vi "PDFCreator Get Options.vi"(0 "PDFCreator._clsPDFCreator":refnum<k7>, 11 "error in (no error)":errorcluster) -> (4 "PDFCreator._clsPDFCreator 2":refnum<k7>, 8 "Options":T1, 15 "error out":errorcluster)   [LabVIEW 2010]
doc: "Jean-Marc Simard \nJanuary 6, 2010"
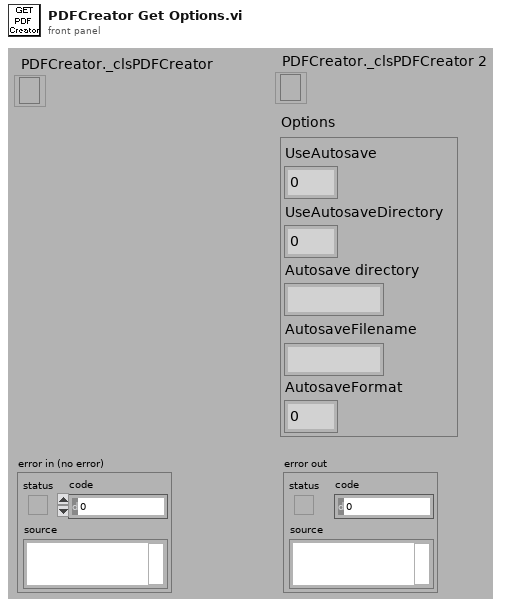
[diagram p1: front panel]
types:
  T1 = cluster{"UseAutosave":i32, "UseAutosaveDirectory":i32, "Autosave directory":string, "AutosaveFilename":string, "AutosaveFormat":i32}
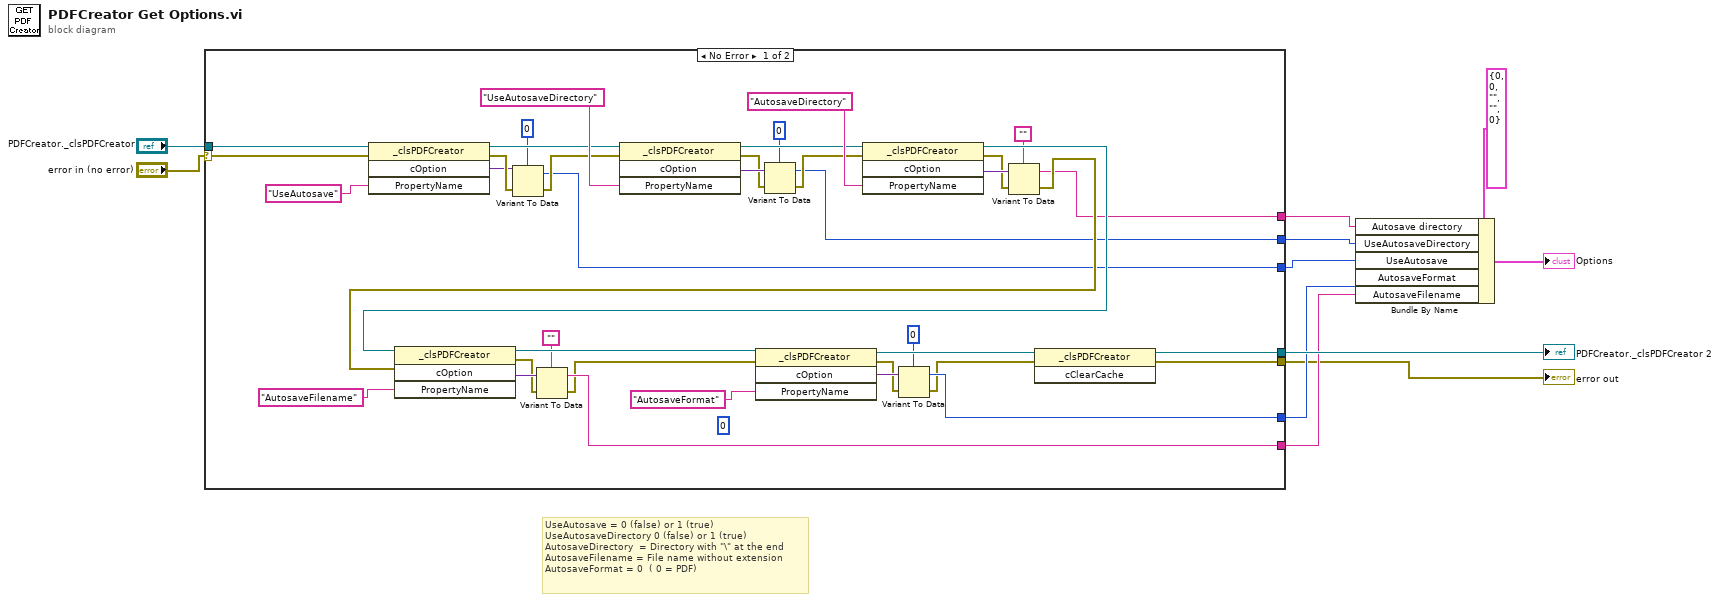
[diagram p0: block diagram]
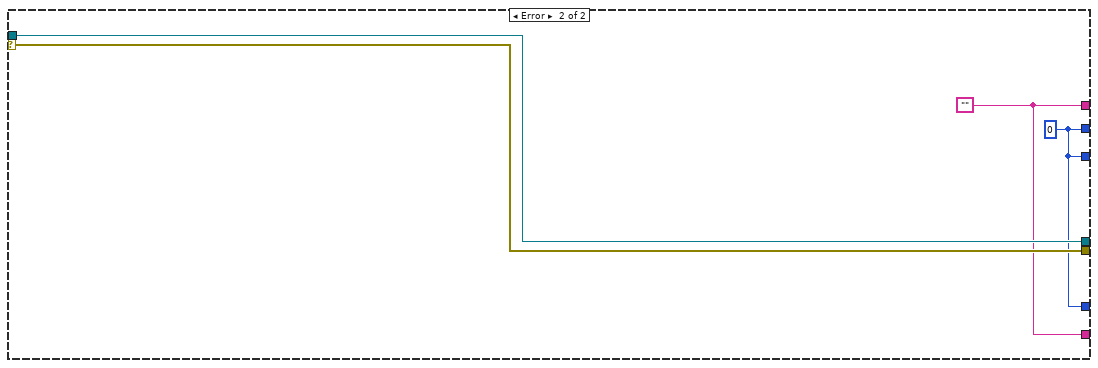
[diagram p2: hidden frame]
diagram:
  # "UseAutosave = 0 (false) or 1 (true)\nUseAutosaveDirectory 0 (false) or 1 (true)\nAutosaveDirectory  = Directory with \"\\\" at the end\nAutosaveFilename = File name without extension \nAutosaveFormat = 0  ( 0 = PDF)"
  n1 = case shown="No Error" "error in (no error)" {
    selector: "error in (no error)" -> [w39 w53]
    tunnel: [w22 w54] -> w11
    tunnel: [w21 w53] -> w1
    tunnel: "PDFCreator._clsPDFCreator" -> [w40 w54]
    tunnel: [w20 w52] -> w9
    tunnel: [w19 w51] -> w8
    tunnel: [w18 w51] -> w7
    tunnel: [w17 w51] -> w6
    tunnel: [w16 w52] -> w5
    frame No Error {
      (unwired) 0
      n2 = invoke class="_clsPDFCreator" method="cOption"(reference=w40, error in=w39, "PropertyName"="UseAutosave") -> (reference out=w48:refnum<k7>, error out=w38:errorcluster, "cOption"=w37:variant)  [unwired: 1 in, 1 out]
      n3 = Variant To Data(error in=w38, Variant=w37, type=0) -> (error out=w35:errorcluster, data=w18:i32)
      n4 = invoke class="_clsPDFCreator" method="cOption"(reference=w48, error in=w35, "PropertyName"="UseAutosaveDirectory") -> (reference out=w46:refnum<k7>, error out=w32:errorcluster, "cOption"=w33:variant)  [unwired: 1 in, 1 out]
      n5 = Variant To Data(error in=w32, Variant=w33, type=0) -> (error out=w31:errorcluster, data=w19:i32)
      n6 = invoke class="_clsPDFCreator" method="cOption"(reference=w46, error in=w31, "PropertyName"="AutosaveDirectory") -> (reference out=w44:refnum<k7>, error out=w28:errorcluster, "cOption"=w29:variant)  [unwired: 1 in, 1 out]
      n7 = Variant To Data(error in=w28, Variant=w29, type="") -> (error out=w27:errorcluster, data=w20:string)
      n8 = invoke class="_clsPDFCreator" method="cOption"(reference=w44, error in=w27, "PropertyName"="AutosaveFilename") -> (reference out=w42:refnum<k7>, error out=w12:errorcluster, "cOption"=w25:variant)  [unwired: 1 in, 1 out]
      n9 = Variant To Data(error in=w12, Variant=w25, type="") -> (error out=w14:errorcluster, data=w16:string)
      n10 = invoke class="_clsPDFCreator" method="cOption"(reference=w42, error in=w14, "PropertyName"="AutosaveFormat") -> (reference out=w41:refnum<k7>, error out=w13:errorcluster, "cOption"=w23:variant)  [unwired: 1 in, 1 out]
      n11 = Variant To Data(error in=w13, Variant=w23, type=0) -> (error out=w15:errorcluster, data=w17:i32)
      n12 = invoke class="_clsPDFCreator" method="cClearCache"(reference=w41, error in=w15) -> (reference out=w22:refnum<k7>, error out=w21:errorcluster)  [unwired: 1 in, 1 out]
    }
    frame Error {
      w51 = 0
      w52 = ""
    }
  }
  "error out" <- w1
  "PDFCreator._clsPDFCreator 2" <- w11
  n13 = Bundle By Name(cluster=T1 {"UseAutosave"=0, "UseAutosaveDirectory"=0, "Autosave directory"="", "AutosaveFilename"="", "AutosaveFormat"=0} ("Options"), "Autosave directory"=w9, "UseAutosaveDirectory"=w8, "UseAutosave"=w7, "AutosaveFormat"=w6, "AutosaveFilename"=w5) -> (→"Options":T1)
